vi "Get Color Ref.vi"(8 "error in (no error)":errorcluster caption="错误输入（无错误）", 11 "Color输入":refnum<class "Color.lvclass">) -> (0 "error out":errorcluster caption="错误输出", 2 "Color":refnum<k24>, 3 "Color输出":refnum<class "Color.lvclass">)   [LabVIEW 2012, in "Color.lvclass"]
uses:
  Color.lvclass
  System.Drawing
  Color.lvclass/Color.ctl
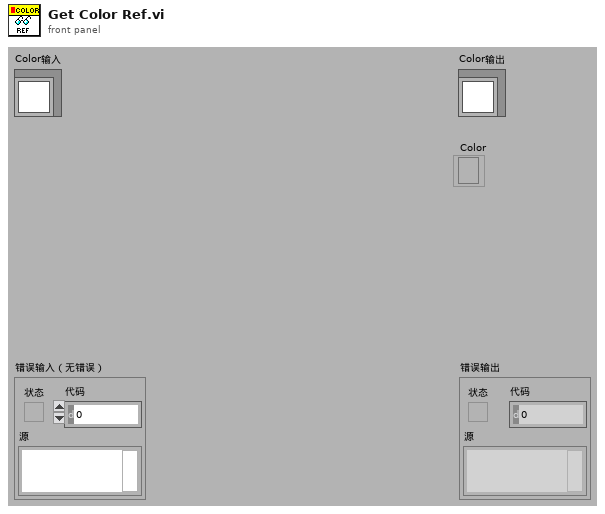
[diagram p1: front panel]
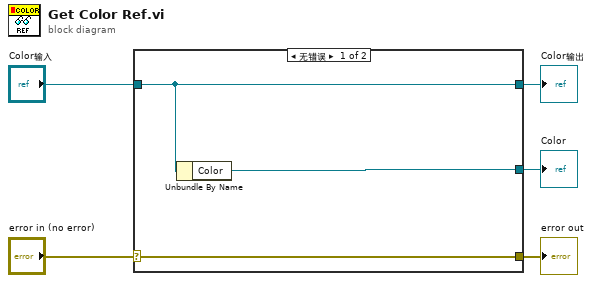
[diagram p0: block diagram]
diagram:
  n1 = case shown="无错误" "error in (no error)" {
    selector: "error in (no error)" -> [w8 w9]
    tunnel: [w8 w9] -> w4
    tunnel: [w7 w10] -> w2
    tunnel: "Color输入" -> [w7 w10]
    tunnel: [w6 _] -> w1
    frame No Error {
      n2 = Unbundle By Name(w7) -> ("Color"=w6:refnum<k24>)
    }
    frame Error {
    }
  }
  "error out" <- w4
  "Color输出" <- w2
  "Color" <- w1
